vi "Vertex.vi"(8 "Index":i32, 10 "Point2D":T1, 11 "DocIn":refnum<k20>) -> (2 "XML":string, 3 "DocOut":refnum<k20>)   [LabVIEW 2014]
uses:
  TypeDefs/Point2DwSlope.ctl
  <resource>/objmgr/DOMUserDefRef.rc
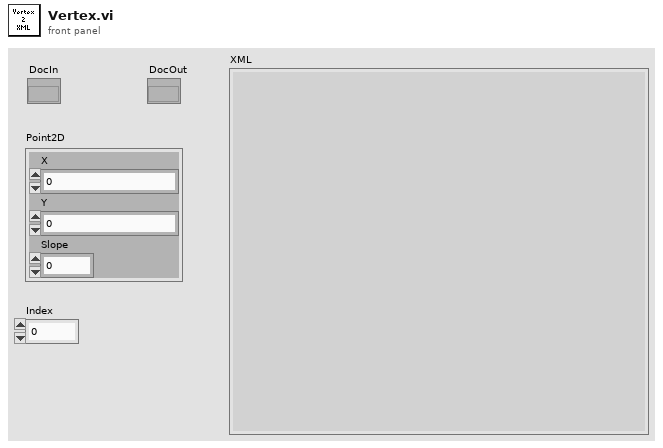
[diagram p1: front panel]
types:
  T1 = typedef "Point2DwSlope.ctl" = cluster{"X":sgl, "Y":sgl, "Slope":dbl}
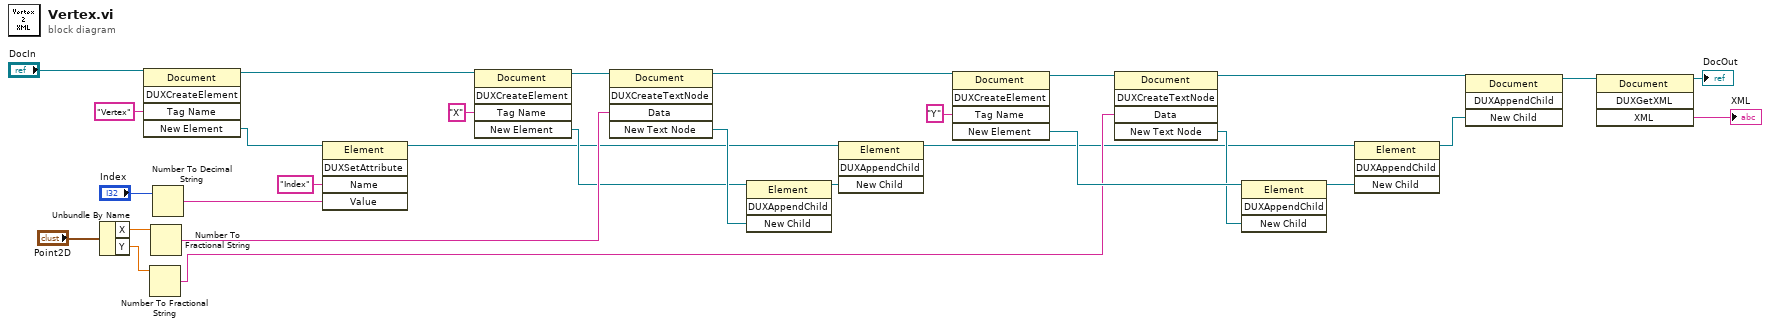
[diagram p0: block diagram]
diagram:
  n1 = Unbundle By Name("Point2D") -> ("X"=w28:sgl, "Y"=w27:sgl)
  n2 = invoke class="Document" method="DUXCreateElement"(reference="DocIn", "Tag Name"="Vertex") -> (reference out=w10:refnum<k20>, "New Element"=w11:refnum<k20>)  [unwired: 3 in, 3 out]
  n3 = Number To Fractional String(number=w27) -> (F-format string=w13:string)  [unwired: 3 in]
  n4 = Number To Fractional String(number=w28) -> (F-format string=w22:string)  [unwired: 3 in]
  n5 = Number To Decimal String(number="Index") -> (decimal integer string=w8:string)  [unwired: 1 in]
  n6 = invoke class="Element" method="DUXSetAttribute"(reference=w11, "Name"="Index", "Value"=w8) -> (reference out=w6:refnum<k20>)  [unwired: 2 in, 4 out]
  n7 = invoke class="Document" method="DUXCreateElement"(reference=w10, "Tag Name"="X") -> (reference out=w23:refnum<k20>, "New Element"=w20:refnum<k20>)  [unwired: 3 in, 3 out]
  n8 = invoke class="Document" method="DUXCreateTextNode"(reference=w23, "Data"=w22) -> (reference out=w15:refnum<k20>, "New Text Node"=w21:refnum<k20>)  [unwired: 3 in, 3 out]
  n9 = invoke class="Element" method="DUXAppendChild"(reference=w20, "New Child"=w21) -> (reference out=w3:refnum<k20>)  [unwired: 2 in, 3 out]
  n10 = invoke class="Element" method="DUXAppendChild"(reference=w6, "New Child"=w3) -> (reference out=w5:refnum<k20>)  [unwired: 2 in, 3 out]
  n11 = invoke class="Document" method="DUXCreateElement"(reference=w15, "Tag Name"="Y") -> (reference out=w17:refnum<k20>, "New Element"=w19:refnum<k20>)  [unwired: 3 in, 3 out]
  n12 = invoke class="Document" method="DUXCreateTextNode"(reference=w17, "Data"=w13) -> (reference out=w14:refnum<k20>, "New Text Node"=w18:refnum<k20>)  [unwired: 3 in, 3 out]
  n13 = invoke class="Element" method="DUXAppendChild"(reference=w19, "New Child"=w18) -> (reference out=w4:refnum<k20>)  [unwired: 2 in, 3 out]
  n14 = invoke class="Element" method="DUXAppendChild"(reference=w5, "New Child"=w4) -> (reference out=w12:refnum<k20>)  [unwired: 2 in, 3 out]
  n15 = invoke class="Document" method="DUXAppendChild"(reference=w14, "New Child"=w12) -> (reference out=w24:refnum<k20>)  [unwired: 2 in, 3 out]
  n16 = invoke class="Document" method="DUXGetXML"(reference=w24) -> (reference out=→"DocOut":refnum<k20>, "XML"=→"XML":string)  [unwired: 3 in, 2 out]
